vi "CreatePrivateEvents.vi"(8 "error in (no error)":errorcluster, 11 "DAQmx":refnum<class "DAQmx.lvclass">) -> (0 "error out":errorcluster, 3 "DAQmx out":refnum<class "DAQmx.lvclass">)   [LabVIEW 2019, in "DAQmx.lvclass"]
uses:
  DAQmx.lvclass
  typedefs/DAQ.Config.AO--Cluster--Array.ctl
  typedefs/DAQ.Config.AO--Cluster.ctl
  typedefs/DAQ.Config.AO.Range--enum.ctl
  typedefs/DAQ.Config.Device Type--enum.ctl
  typedefs/DAQ.Config.AI--Cluster--Array.ctl
  typedefs/DAQ.Config.AI--Cluster.ctl
  typedefs/DAQ.Config.AI.Coupling--enum.ctl
  typedefs/DAQ.Config.AI.Range--enum.ctl
  typedefs/DAQ.Config.Timing--Cluster.ctl
  typedefs/DAQ.Config.Timing.Sampling--Cluster.ctl
  typedefs/Message--Cluster.ctl
  typedefs/DAQmx.Commands--enum.ctl
  DAQmx.lvclass/DAQmx.ctl
  <vilib>/JKI/JKI SMO/SMO/SMO.lvclass
panel:
  # "For instructions on how to use the JKI State Machine Objects, examples and video tutorials, visit:\nhttp://jki.net/state-machine-objects/\n\nJKI State Machine Objects™\nhttp://jki.net/state-machine-objects/\nCopyright (C) 2005-2015, JKI <info@jki.net>\nALL RIGHTS RESERVED"
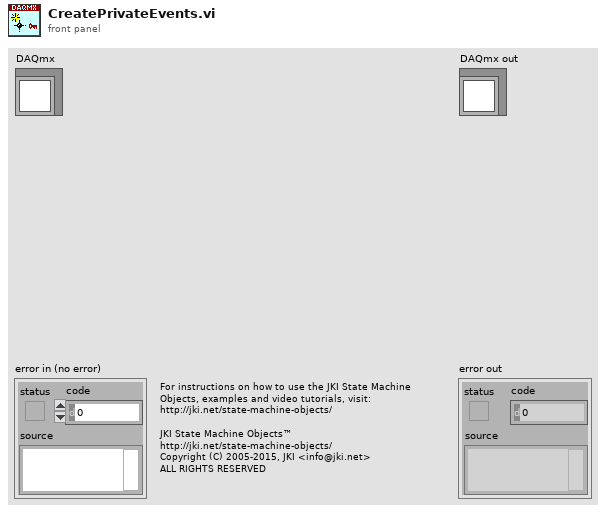
[diagram p1: front panel]
types:
  T1 = typedef "DAQmx.lvclass/Message--Cluster.ctl" = cluster{"command":T2, "Argument":string}
  T2 = typedef "DAQmx.lvclass/DAQmx.Commands--enum.ctl" = enum16{"idle", "start", "stop", "calibrate", "auto", "exit"}
  T3 = typedef "DAQmx.lvclass/DAQ.Config.Timing--Cluster.ctl" = cluster{"Sampling":T4, "Fs_Out":dbl}
  T4 = typedef "DAQmx.lvclass/DAQ.Config.Timing.Sampling--Cluster.ctl" = cluster{"Fs":dbl, "#s":i32}
  T5 = typedef "DAQmx.lvclass/DAQ.Config.AI--Cluster--Array.ctl" = T6[]
  T6 = typedef "DAQmx.lvclass/DAQ.Config.AI--Cluster.ctl" = cluster{"Channels":tag, "Coupling":T7, "Range":T8, "input terminal configuration":i32, "Type":T9}
  T7 = typedef "DAQmx.lvclass/DAQ.Config.AI.Coupling--enum.ctl" = u16
  T8 = typedef "DAQmx.lvclass/DAQ.Config.AI.Range--enum.ctl" = enum16{"±0.316", "±1.00", "±3.16", "±10.0", "±31.6", "±42.4", ""}
  T9 = typedef "DAQmx.lvclass/DAQ.Config.Device Type--enum.ctl" = enum16{"None", "USB-4431", "PXI-446x"}
  T10 = typedef "DAQmx.lvclass/DAQ.Config.AO--Cluster--Array.ctl" = T11[]
  T11 = typedef "DAQmx.lvclass/DAQ.Config.AO--Cluster.ctl" = cluster{"Channels":tag, "Range":T12, "output terminal configuration":i32, "Type":T9}
  T12 = typedef "DAQmx.lvclass/DAQ.Config.AO.Range--enum.ctl" = enum16{"±0.1", "±1.0", "±3.5", "±10.0", ""}
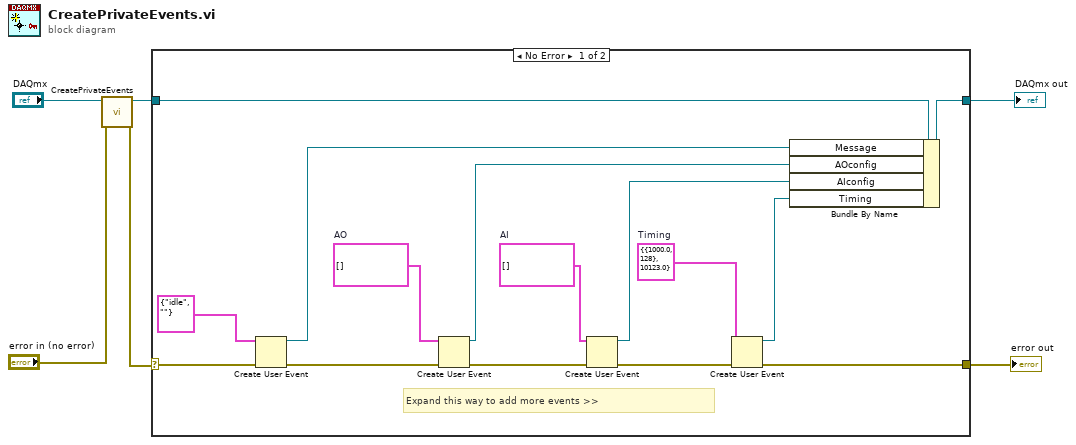
[diagram p0: block diagram]
diagram:
  n1 = call-parent "CreatePrivateEvents.vi"("error in (no error)"="error in (no error)", "SMO"="DAQmx") -> ("error out"=w4:errorcluster, "SMO out"=w5:refnum<class "DAQmx.lvclass">)  [unwired: 8 in]
  n2 = case shown="No Error" w4 {
    selector: w4 -> [w15 w23]
    tunnel: [w9 w23] -> w2
    tunnel: [w20 w22] -> w3
    tunnel: w5 -> [w21 w22]
    frame No Error {
      w8 = T3 {"Sampling"={"Fs"=1000.0, "#s"=128}, "Fs_Out"=10123.0}  # Timing
      w18 = T5 []  # AI
      w19 = T10 []  # AO
      # "Expand this way to add more events >>"
      n3 = Create User Event(user event datatype=T1 {"command"=enum."idle", "Argument"=""} ("Message"), error in=w15) -> (user event=w13:refnum<user-event>, error out=w14:errorcluster)
      n4 = Create User Event(user event datatype=w19, error in=w14) -> (user event=w12:refnum<user-event>, error out=w17:errorcluster)
      n5 = Create User Event(user event datatype=w18, error in=w17) -> (user event=w11:refnum<user-event>, error out=w16:errorcluster)
      n6 = Create User Event(user event datatype=w8, error in=w16) -> (user event=w10:refnum<user-event>, error out=w9:errorcluster)
      n7 = Bundle By Name(cluster=w21, "Message"=w13, "AOconfig"=w12, "AIconfig"=w11, "Timing"=w10) -> (w20:refnum<class "DAQmx.lvclass">)
    }
    frame Error {
    }
  }
  "error out" <- w2
  "DAQmx out" <- w3
